vi "test_Loop OpenClose (Session).vi"() -> ()   [LabVIEW 2020]
uses:
  <instrlib>/AIM GmbH/_AIM 664/bsp/Fdx Create Session (Tx-UDP Port-Oriented).vi
  <instrlib>/AIM GmbH/_AIM 664/bsp/Fdx Create Session (Rx-VL-Oriented).vi
  <instrlib>/AIM GmbH/_AIM 664/AIM664LV.lvlib
panel:
  in  "simulate execution time mS 2":u32=10
  in  "board 2":u32
  in  "port 2":u32
  in  "port":u32
  in  "board":u32
  in  "simulate execution time mS":u32=10
  in  "idle before iterations mS":u32=1000
  out "error out":errorcluster
  out "executed":i32
  in  "Iterations":i32=1
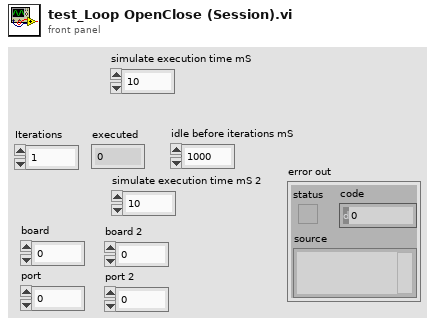
[diagram p1: front panel]
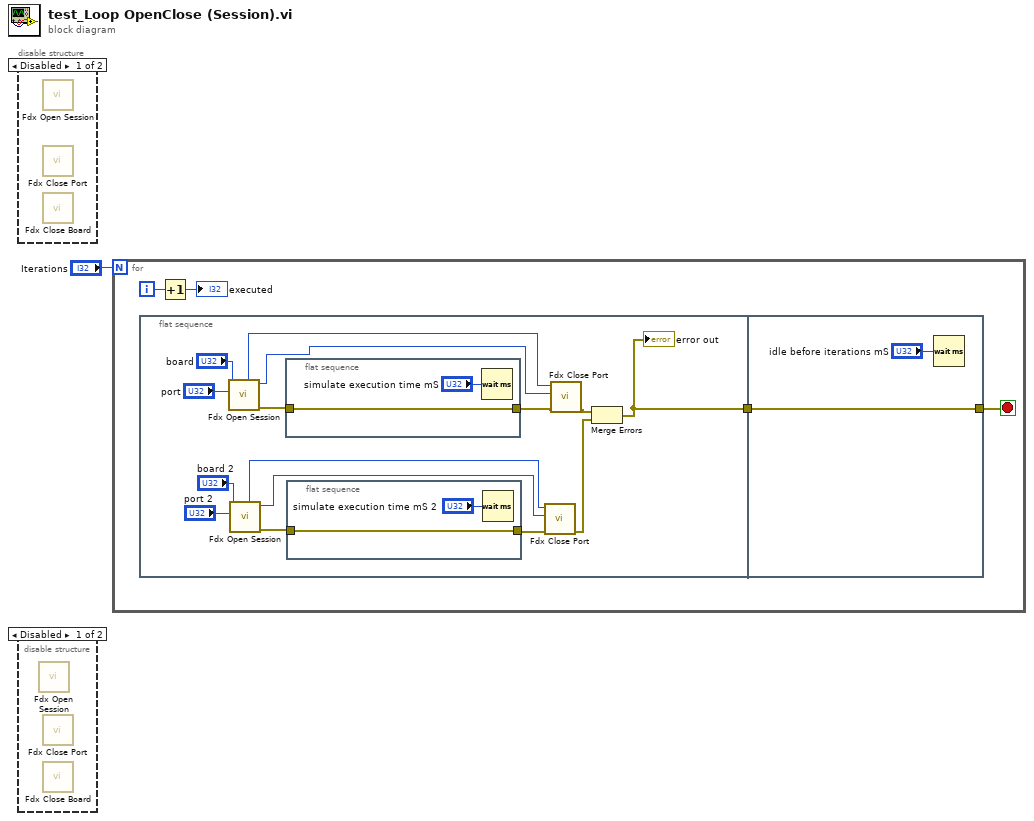
[diagram p0: block diagram]
diagram:
  n1 = disable-structure shown="Disabled" {
    frame Disabled {
      n2 = call-poly <instrlib>:"Fdx Open Session.vi"() -> ()  [unwired: 7 in, 5 out]
      n3 = call <instrlib>:"Fdx Close Port.vi"() -> ()  [unwired: 10 in, 2 out]
      n4 = call <instrlib>:"Fdx Close Board.vi"() -> ()  [unwired: 11 in, 1 out]
    }
    frame Enabled {
    }
  }
  n5 = disable-structure shown="Disabled" {
    frame Disabled {
      n6 = call-poly <instrlib>:"Fdx Open Session.vi"() -> ()  [unwired: 7 in, 5 out]
      n7 = call <instrlib>:"Fdx Close Port.vi"() -> ()  [unwired: 10 in, 2 out]
      n8 = call <instrlib>:"Fdx Close Board.vi"() -> ()  [unwired: 11 in, 1 out]
    }
    frame Enabled {
    }
  }
  n9 = for {
    N: "Iterations" -> [_]
    i -> [w3]
    stop <- w5 stop-if-true
    n10 = flat-sequence {
      tunnel: [w13] -> w4
      tunnel: [w25] -> w5
      tunnel: w4 -> [w25]
      frame #0 {
        n11 = call-poly <instrlib>:"Fdx Open Session.vi"("port"="port", "board"="board") -> ("error out"=w20:errorcluster, "port handle out"=w14:u32, "InstrumentHandle_board out"=w15:u32)  [unwired: 5 in, 2 out]
        n12 = call-poly <instrlib>:"Fdx Open Session.vi"("port"="port 2", "board"="board 2") -> ("error out"=w10:errorcluster, "InstrumentHandle_port out"=w6:u32, "InstrumentHandle_board out"=w7:u32)  [unwired: 4 in, 3 out]
        n13 = flat-sequence {
          tunnel: w20 -> [w24]
          tunnel: [w24] -> w19
          frame #0 {
            n14 = Wait (ms)(milliseconds to wait="simulate execution time mS") -> ()  [unwired: 1 out]
          }
        }
        n15 = flat-sequence {
          tunnel: w10 -> [w22]
          tunnel: [w22] -> w9
          frame #0 {
            n16 = Wait (ms)(milliseconds to wait="simulate execution time mS 2") -> ()  [unwired: 1 out]
          }
        }
        n17 = call <instrlib>:"Fdx Close Port.vi"("error in"=w9, "InstrumentHandle_port in"=w6, "InstrumentHandle_board in"=w7) -> ("error out"=w8:errorcluster)  [unwired: 7 in, 1 out]
        n18 = call <instrlib>:"Fdx Close Port.vi"("error in"=w19, "InstrumentHandle_port in"=w14, "InstrumentHandle_board in"=w15) -> ("error out"=w18:errorcluster)  [unwired: 7 in, 1 out]
        n19 = Merge Errors(w18, w8) -> (w13:errorcluster)
        "error out" <- w13
      }
      frame #1 {
        n20 = Wait (ms)(milliseconds to wait="idle before iterations mS") -> ()  [unwired: 1 out]
      }
    }
    n21 = Increment(x=w3) -> (x+1=→"executed":i32)
  }
